vi "Calculate.vi"(7 "Measurement path in":path=path "D:/martin/WAC/WACsw - github/control_software/Filter function meter/Template/Example of FF meter template_data/FF_calibration_template_line_0010/session.info", 8 "error in (no error)":errorcluster, 11 "GOLPI ref. in":T1={"pipe handle"={"lv_proc.dll file path"=path "", "process instance handle"=[], "debug mode"=FALSE, "debug data"=[]}, "fast read timeout [ms]"=500, "fast read settle time [ms]"=10, "fast read to multiple [ms]"=1, "max elements per input line"=100, "slow read timeout [ms]"=5000, "stdin double format specifier"="%_16e", "max elements per stdout output column"=100, "console mode bitstream"=FALSE, "bitstream first read timeout [ms]"=1000, "bitstream read timeout [ms]"=50, "struct transfer possible"=FALSE, "matlab mode"=FALSE}) -> (0 "error out":errorcluster, 3 "GOLPI ref. out":T1={"pipe handle"={"lv_proc.dll file path"=path "", "process instance handle"=[], "debug mode"=FALSE, "debug data"=[]}, "fast read timeout [ms]"=500, "fast read settle time [ms]"=10, "fast read to multiple [ms]"=1, "max elements per input line"=100, "slow read timeout [ms]"=5000, "stdin double format specifier"="%_16e", "max elements per stdout output column"=100, "console mode bitstream"=FALSE, "bitstream first read timeout [ms]"=1000, "bitstream read timeout [ms]"=50, "struct transfer possible"=FALSE, "matlab mode"=FALSE})   [LabVIEW 2020]
doc: "Starts and waits for QWTB calculation."
uses:
  external libraries/GOLPI 0.7.3.1 source distribution LV 20.0 32 bit/GOLPI reference Type Def.ctl
  external libraries/GOLPI 0.7.3.1 source distribution LV 20.0 32 bit/Pipe Handle.ctl
  external libraries/GOLPI 0.7.3.1 source distribution LV 20.0 32 bit/GOLPI library.lvlib
  external libraries/GOLPI 0.7.3.1 source distribution LV 20.0 32 bit/LV Process library.lvlib
panel:
  out "command\n(for debug)":string="addpath('info'); addpath('qwtb'); qwtb_exec_algorithm('%s', 0, 1); disp('FINISHEDCR')"
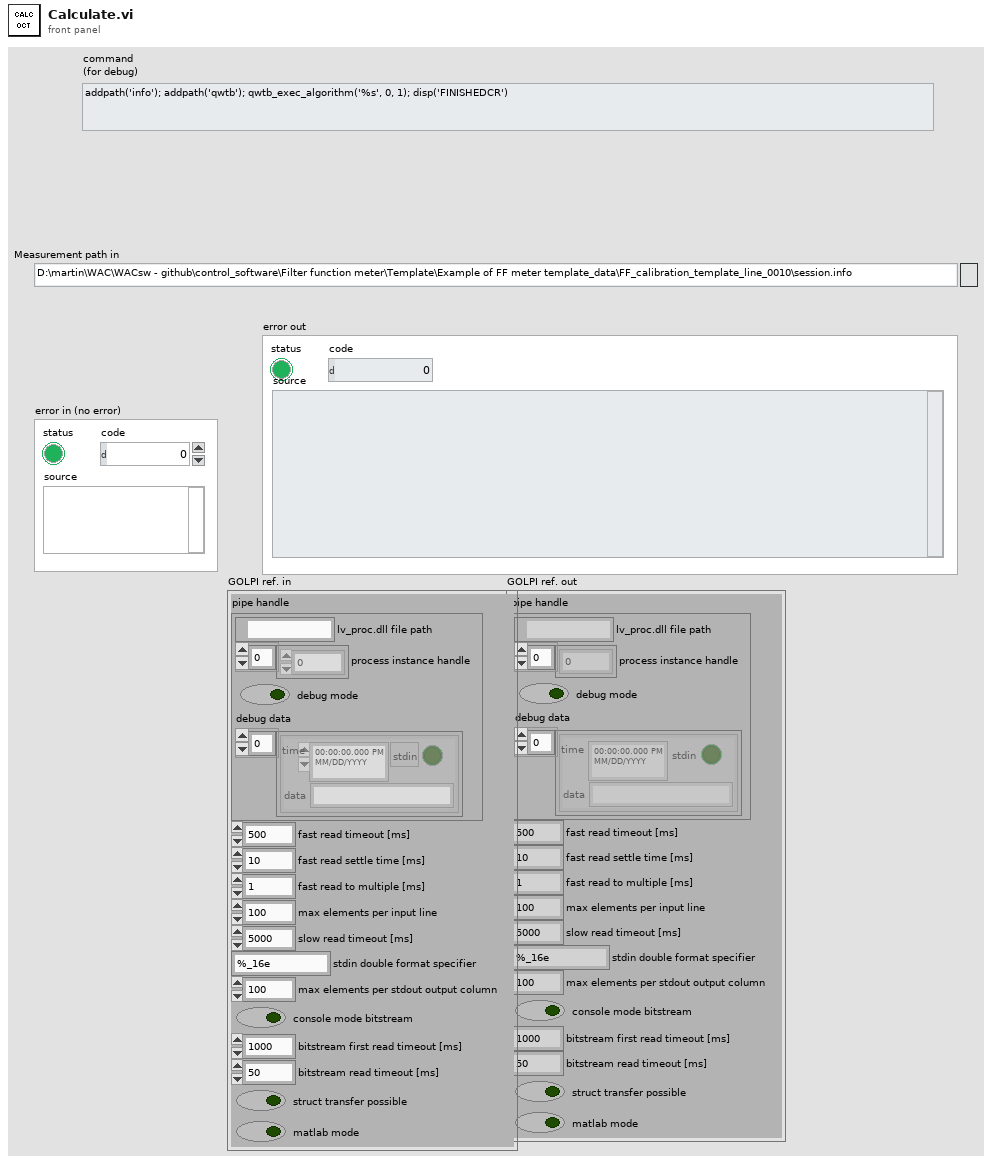
[diagram p1: front panel]
types:
  T1 = typedef "GOLPI library.lvlib/GOLPI reference Type Def.ctl" = cluster{"pipe handle":T2, "fast read timeout [ms]":u32, "fast read settle time [ms]":u32, "fast read to multiple [ms]":u32, "max elements per input line":u32, "slow read timeout [ms]":u32, "stdin double format specifier":string, "max elements per stdout output column":u32, "console mode bitstream":bool, "bitstream first read timeout [ms]":u32, "bitstream read timeout [ms]":u32, "struct transfer possible":bool, "matlab mode":bool}
  T2 = typedef "LV Process library.lvlib/Pipe Handle.ctl" = cluster{"lv_proc.dll file path":path, "process instance handle":u32[], "debug mode":bool, "debug data":cluster{"time":timestamp, "stdin":bool, "data":string}[]}
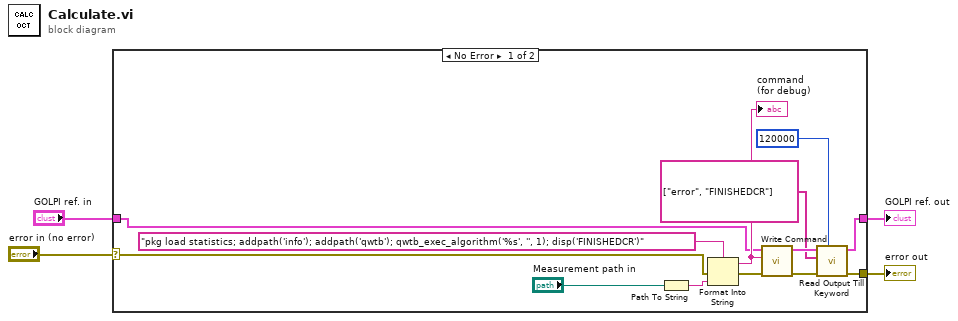
[diagram p0: block diagram]
diagram:
  n1 = case shown="No Error" "error in (no error)" {
    selector: "error in (no error)" -> [w5 w19]
    tunnel: [w8 w19] -> w4
    tunnel: [w7 w18] -> w3
    tunnel: "GOLPI ref. in" -> [w6 w18]
    frame No Error {
      n2 = Path To String(path="Measurement path in") -> (string=w15:string)
      n3 = Format Into String(format string="pkg load statistics; addpath('info'); addpath('qwtb'); qwtb_exec_algorithm('%s', '', 1); disp('FINISHEDCR')", error in=w5, w15) -> (resulting string=w9:string, error out=w14:errorcluster)  [unwired: 1 in]
      "command\n(for debug)" <- w9
      n4 = call "Write Command.vi"("error in"=w14, "command"=w9, "GOLPI ref. in"=w6) -> ("error out"=w13:errorcluster, "GOLPI ref. out"=w12:T1)  [unwired: 7 in]
      n5 = call "Read Output Till Keyword.vi"("timeout [ms]"=u32 120000, "error in"=w13, "keywords"=string[] ["error", "FINISHEDCR"], "GOLPI ref. in"=w12) -> ("error out"=w8:errorcluster, "GOLPI ref. out"=w7:T1)  [unwired: 4 in, 2 out]
    }
    frame Error {
    }
  }
  "error out" <- w4
  "GOLPI ref. out" <- w3
